vi "ANDOR_Init.vi"(8 "error in (no error)":errorcluster) -> (0 "error out":errorcluster, 2 "Camera Capabilities":T1, 3 "Camera Parameters":T2)   [LabVIEW 2010]
uses:
  <userlib>/_andor/atmcd32d.llb/AndorCapabilities typedef.ctl
  <userlib>/_andor/atmcd32d.llb/Error Code Enum typedef.ctl
  <userlib>/_andor/atmcd32d.llb/HSSpeed_type typedef.ctl
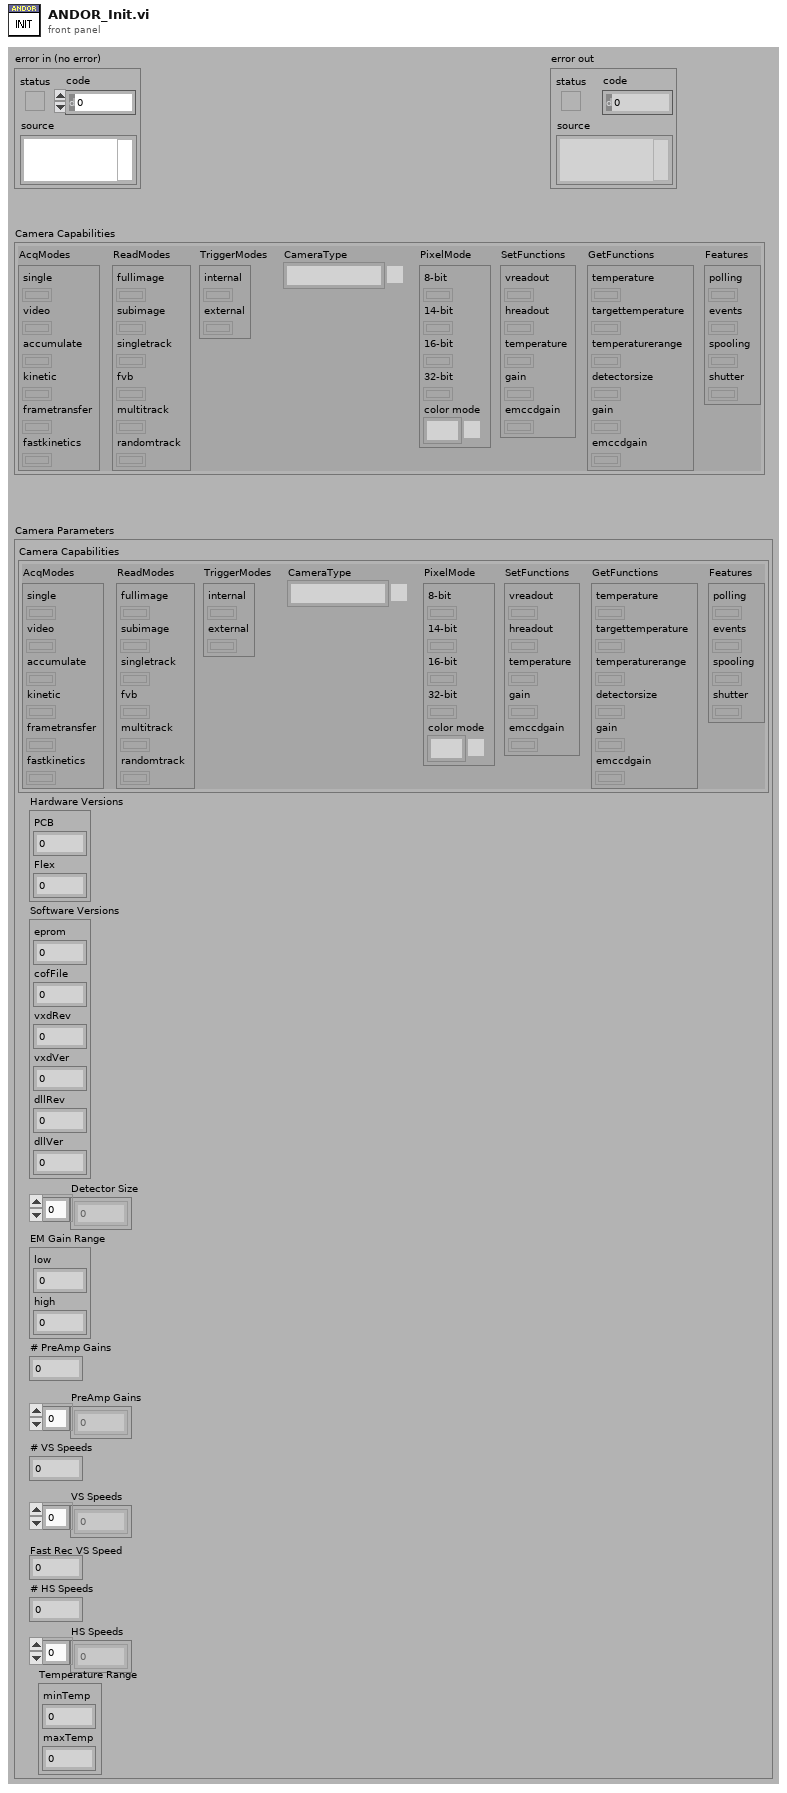
[diagram p1: front panel]
types:
  T1 = typedef "AndorCapabilities typedef.ctl" = cluster{"AcqModes":cluster{"single":bool, "video":bool, "accumulate":bool, "kinetic":bool, "frametransfer":bool, "fastkinetics":bool}, "ReadModes":cluster{"fullimage":bool, "subimage":bool, "singletrack":bool, "fvb":bool, "multitrack":bool, "randomtrack":bool}, "TriggerModes":cluster{"internal":bool, "external":bool}, "CameraType":enum32{"PDA", "iXon", "ICCD", "EMCCD", "CCD", "iStar", "third party camera"}, "PixelMode":cluster{"8-bit":bool, "14-bit":bool, "16-bit":bool, "32-bit":bool, "color mode":enum16{"Mono", "RGB", "CMY"}}, "SetFunctions":cluster{"vreadout":bool, "hreadout":bool, "temperature":bool, "gain":bool, "emccdgain":bool}, "GetFunctions":cluster{"temperature":bool, "targettemperature":bool, "temperaturerange":bool, "detectorsize":bool, "gain":bool, "emccdgain":bool}, "Features":cluster{"polling":bool, "events":bool, "spooling":bool, "shutter":bool}}
  T2 = cluster{"Camera Capabilities":T1, "Hardware Versions":cluster{"PCB":u32, "Flex":u32}, "Software Versions":cluster{"eprom":u32, "cofFile":u32, "vxdRev":u32, "vxdVer":u32, "dllRev":u32, "dllVer":u32}, "Detector Size":i32[], "EM Gain Range":cluster{"low":i32, "high":i32}, "# PreAmp Gains":i32, "PreAmp Gains":sgl[], "# VS Speeds":i32, "VS Speeds":sgl[], "Fast Rec VS Speed":i32, "# HS Speeds":i32, "HS Speeds":sgl[], "Temperature Range":cluster{"minTemp":i32, "maxTemp":i32}}
  T3 = typedef "Error Code Enum typedef.ctl" = enum32{"N/A (0)", "DRV_ERROR_CODES", "DRV_SUCCESS", "DRV_VXDNOTINSTALLED", "DRV_ERROR_SCAN", "DRV_ERROR_CHECK_SUM", "DRV_ERROR_FILELOAD", "DRV_UNKNOWN_FUNC", "DRV_ERROR_VXD_INIT", "DRV_ERROR_ADDRESS", "DRV_ERROR_PAGELOCK", "DRV_ERROR_PAGEUNLOCK", "DRV_ERROR_BOARDTEST", "DRV_ERROR_ACK", "DRV_ERROR_UP_FIFO", "DRV_ERROR_PATTERN", "N/A (16)", "DRV_ACQUISITION_ERRORS", "DRV_ACQ_BUFFER", "DRV_ACQ_DOWNFIFO_FULL", "DRV_PROC_UNKONWN_INSTRUCTION", "DRV_ILLEGAL_OP_CODE", "DRV_KINETIC_TIME_NOT_MET", "DRV_ACCUM_TIME_NOT_MET", "DRV_NO_NEW_DATA", "N/A (25)", "DRV_SPOOLERROR", "N/A (27)", "N/A (28)", "N/A (29)", "N/A (30)", "N/A (31)", "N/A (32)", "DRV_TEMPERATURE_CODES", "DRV_TEMPERATURE_OFF", "DRV_TEMPERATURE_NOT_STABILIZED", "DRV_TEMPERATURE_STABILIZED", "DRV_TEMPERATURE_NOT_REACHED", "DRV_TEMPERATURE_OUT_RANGE", "DRV_TEMPERATURE_NOT_SUPPORTED", "DRV_TEMPERATURE_DRIFT", "N/A (41)", "N/A (42)", "N/A (43)", "N/A (44)", "N/A (45)", "N/A (46)", "N/A (47)", "N/A (48)", "DRV_GENERAL_ERRORS", "DRV_INVALID_AUX", "DRV_COF_NOTLOADED", "DRV_FPGAPROG", "DRV_FLEXERROR", "DRV_GPIBERROR", "N/A (55)", "N/A (56)", "N/A (57)", "N/A (58)", "N/A (59)", "N/A (60)", "N/A (61)", "N/A (62)", "N/A (63)", "DRV_DATATYPE", "DRV_DRIVER_ERRORS", "DRV_P1INVALID", "DRV_P2INVALID", "DRV_P3INVALID", "DRV_P4INVALID", "DRV_INIERROR", "DRV_COFERROR", "DRV_ACQUIRING", "DRV_IDLE", "DRV_TEMPCYCLE", "DRV_NOT_INITIALIZED", "DRV_P5INVALID", "DRV_P6INVALID", "DRV_INVALID_MODE", "DRV_INVALID_FILTER", "DRV_I2CERRORS", "DRV_I2CDEVNOTFOUND", "DRV_I2CTIMEOUT", "DRV_P7INVALID", "N/A (84)", "N/A (85)", "N/A (86)", "N/A (87)", "N/A (88)", "N/A (89)", "DRV_IOCERROR", "DRV_VRMVERSIONERROR"}
  T4 = typedef "HSSpeed_type typedef.ctl" = enum16{"EM Amp", "Conventional Amp"}
  T5 = cluster{"eprom":u32, "cofFile":u32, "vxdRev":u32, "vxdVer":u32, "dllRev":u32, "dllVer":u32}
  T6 = cluster{"caps":T1, "Hardware Versions":cluster{"PCB":u32, "Flex":u32}, "Software Versions":cluster{"eprom":u32, "cofFile":u32, "vxdRev":u32, "vxdVer":u32, "dllRev":u32, "dllVer":u32}, "Detector Size":i32[], "EM Gain Range":cluster{"low":i32, "high":i32}, "number":i32, sgl[], "number":i32, sgl[], "index":u32, "number":i32, sgl[], "Temperature Range":cluster{"minTemp":i32, "maxTemp":i32}}
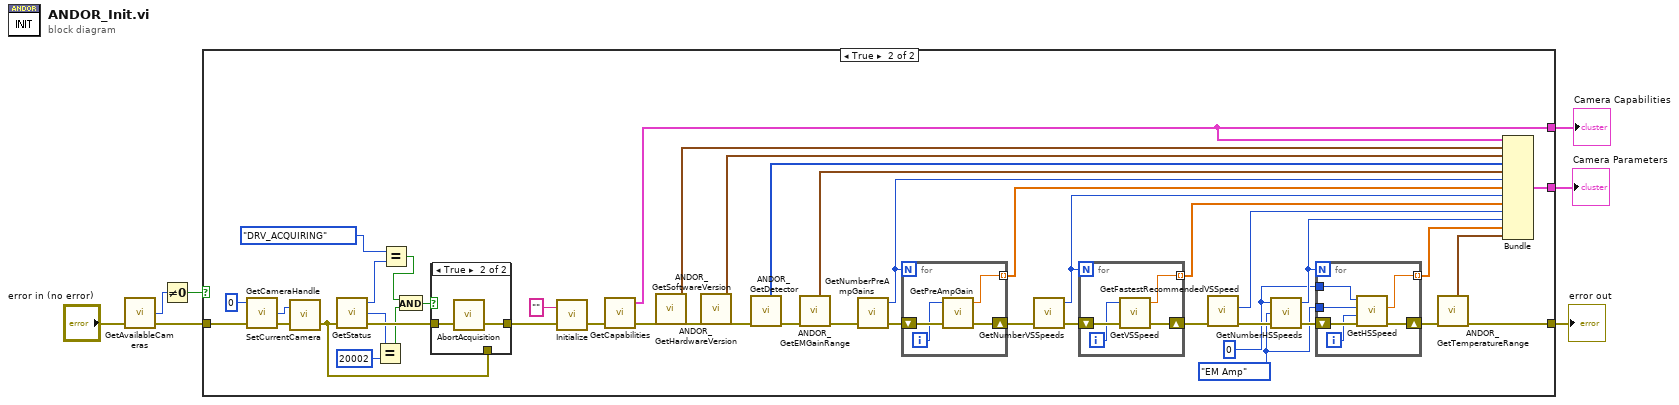
[diagram p0: block diagram]
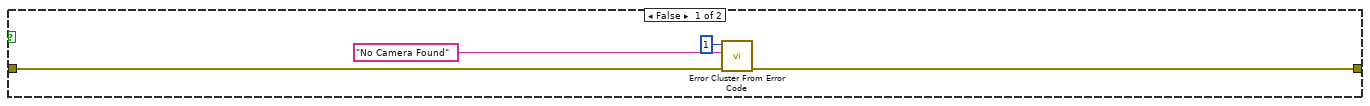
[diagram p2: hidden frame]
diagram:
  n1 = call <userlib>:"GetAvailableCameras.vi"("error in (no error)"="error in (no error)") -> ("error out"=w6:errorcluster, "totalCameras"=w4:i32)  [unwired: 2 in, 1 out]
  n2 = Not Equal To 0?(x=w4) -> (x != 0?=w5:bool)
  n3 = case shown="True" w5 {
    tunnel: [w10 w24] -> w7
    tunnel: w6 -> [w11 w22]
    tunnel: [_ w43] -> w2
    tunnel: [_ w28] -> w1
    frame False {
      n4 = call <vilib>:"Error Cluster From Error Code.vi"("error in (no error)"=w11, "error message (\"\")"="No Camera Found" ("error message (\"\")"), "error code (0)"=1) -> ("error out"=w10:errorcluster)  [unwired: 6 in]
    }
    frame True {
      w26 = HSSpeed_type_typedef."EM Amp" ("type")
      w27 = 0 ("channel")
      n5 = call <userlib>:"GetCameraHandle.vi"("error in (no error)"=w22, "cameraIndex"=0) -> ("error out"=w55:errorcluster, "cameraHandle"=w54:i32)  [unwired: 1 in, 1 out]
      n6 = call <userlib>:"SetCurrentCamera.vi"("error in (no error)"=w55, "cameraHandle"=w54) -> ("error out"=w13:errorcluster)  [unwired: 1 out]
      n7 = call <userlib>:"GetStatus.vi"("error in (no error)"=w13) -> ("error out"=w21:errorcluster, "DLL error code"=w17:u32, "status"=w19:T3)  [unwired: 2 in]
      n8 = Equal?(x=w17, y=u32 20002) -> (x = y?=w15:bool)
      n9 = Equal?(x=Error_Code_Enum_typedef."DRV_ACQUIRING" ("status"), y=w19) -> (x = y?=w14:bool)
      n10 = And(x=w14, y=w15) -> (x .and. y?=w12:bool)
      n11 = case shown="True" w12 {
        tunnel: w21 -> [_ w59]
        tunnel: [w57 w58] -> w20
        tunnel: w13 -> [w57 _]
        frame False {
        }
        frame True {
          n12 = call <userlib>:"AbortAcquisition.vi"("error in (no error)"=w59) -> ("error out"=w58:errorcluster)  [unwired: 1 in, 1 out]
        }
      }
      n13 = call <userlib>:"Initialize.vi"("error in (no error)"=w20, "directory (\"\")"="" ("directory (\"\")")) -> ("error out"=w52:errorcluster)  [unwired: 1 out]
      n14 = call <userlib>:"GetCapabilities.vi"("error in (no error)"=w52) -> ("error out"=w51:errorcluster, "caps"=w43:T1)  [unwired: 2 in, 1 out]
      n15 = call "ANDOR_GetHardwareVersion.vi"("error in (no error)"=w51) -> ("Hardware Versions"=w42:cluster{"PCB":u32, "Flex":u32}, "error out"=w50:errorcluster)  [unwired: 18 in, 7 out]
      n16 = call "ANDOR_GetSoftwareVersion.vi"("error in (no error)"=w50) -> ("Software Versions"=w41:T5, "error out"=w49:errorcluster)  [unwired: 18 in, 7 out]
      n17 = call "ANDOR_GetDetector.vi"("error in (no error)"=w49) -> ("error out"=w46:errorcluster, "Detector Size"=w40:i32[])  [unwired: 6 in, 3 out]
      n18 = call "ANDOR_GetEMGainRange.vi"("error in (no error)"=w46) -> ("error out"=w48:errorcluster, "EM Gain Range"=w39:cluster{"low":i32, "high":i32})  [unwired: 6 in, 3 out]
      n19 = call <userlib>:"GetNumberPreAmpGains.vi"("error in (no error)"=w48) -> ("error out"=w47:errorcluster, "number"=w38:i32)  [unwired: 2 in, 1 out]
      n20 = for {
        N: w38 -> [_]
        shift-right: [w72] -> w45
        shift-left: w47 -> [w73]
        tunnel: [w70] -> w37 mode=indexing
        i -> [w71]
        n21 = call <userlib>:"GetPreAmpGain.vi"("error in (no error)"=w73, "index"=w71) -> ("error out"=w72:errorcluster, "gain"=w70:sgl)  [unwired: 1 in, 1 out]
      }
      n22 = call <userlib>:"GetNumberVSSpeeds.vi"("error in (no error)"=w45) -> ("error out"=w44:errorcluster, "number"=w36:i32)  [unwired: 2 in, 1 out]
      n23 = for {
        N: w36 -> [_]
        shift-right: [w68] -> w34
        shift-left: w44 -> [w69]
        tunnel: [w66] -> w35 mode=indexing
        i -> [w67]
        n24 = call <userlib>:"GetVSSpeed.vi"("error in (no error)"=w69, "index"=w67) -> ("error out"=w68:errorcluster, "speed"=w66:sgl)  [unwired: 1 in, 1 out]
      }
      n25 = call <userlib>:"GetFastestRecommendedVSSpeed.vi"("error in (no error)"=w34) -> ("error out"=w32:errorcluster, "index"=w33:u32)  [unwired: 3 in, 2 out]
      n26 = call <userlib>:"GetNumberHSSpeeds.vi"("error in (no error)"=w32, "type"=w26, "channel"=w27) -> ("error out"=w31:errorcluster, "number"=w30:i32)  [unwired: 1 out]
      n27 = for {
        N: w30 -> [_]
        shift-right: [w64] -> w25
        shift-left: w31 -> [w65]
        tunnel: [w62] -> w29 mode=indexing
        tunnel: w27 -> [w61]
        tunnel: w26 -> [w60]
        i -> [w63]
        n28 = call <userlib>:"GetHSSpeed.vi"("error in (no error)"=w65, "index"=w63, "type"=w60, "channel"=w61) -> ("error out"=w64:errorcluster, "speed"=w62:sgl)  [unwired: 1 in, 1 out]
      }
      n29 = call "ANDOR_GetTemperatureRange.vi"("error in (no error)"=w25) -> ("error out"=w24:errorcluster, "Temperature Range"=w23:cluster{"minTemp":i32, "maxTemp":i32})  [unwired: 6 in, 3 out]
      n30 = Bundle("caps"=w43, "Hardware Versions"=w42, "Software Versions"=w41, "Detector Size"=w40, "EM Gain Range"=w39, "number"=w38, w37, "number"=w36, w35, "index"=w33, "number"=w30, w29, "Temperature Range"=w23) -> (w28:T6)  [unwired: 1 in]
    }
  }
  "error out" <- w7
  "Camera Capabilities" <- w2
  "Camera Parameters" <- w1
